vi "GS Var Common Ana Fixed Settings.vi"(1 "Action(GET)":enum16{"GET", "SET"}(ring), 7 "Common Analog Var Fixed in":T4[](array[typedef]) {"Default Scaling"."Offset" format="%.5f"; "Default Scaling"."Gain" format="%.5f"}, 9 "Common Digital Var Fixed in":T1[](array[typedef]), 11 "error in (no error)":errorcluster) -> (8 "Common Analog Var Fixed out":T4[](array[typedef]) {"Default Scaling"."Offset" format="%.5f"; "Default Scaling"."Gain" format="%.5f"}, 10 "Common Digital var Fixed":T1[](array[typedef]), 15 "error out":errorcluster)   [LabVIEW 2011]
uses:
  Fixed Analog Channel Definition.ctl
  Units/Quantity enum.ctl
  Update frequensies.ctl
  Channel catagory Enum.ctl
  Scaling.ctl
  Channel Classification Enum.ctl
  Fixed Digital Channel Definition.ctl
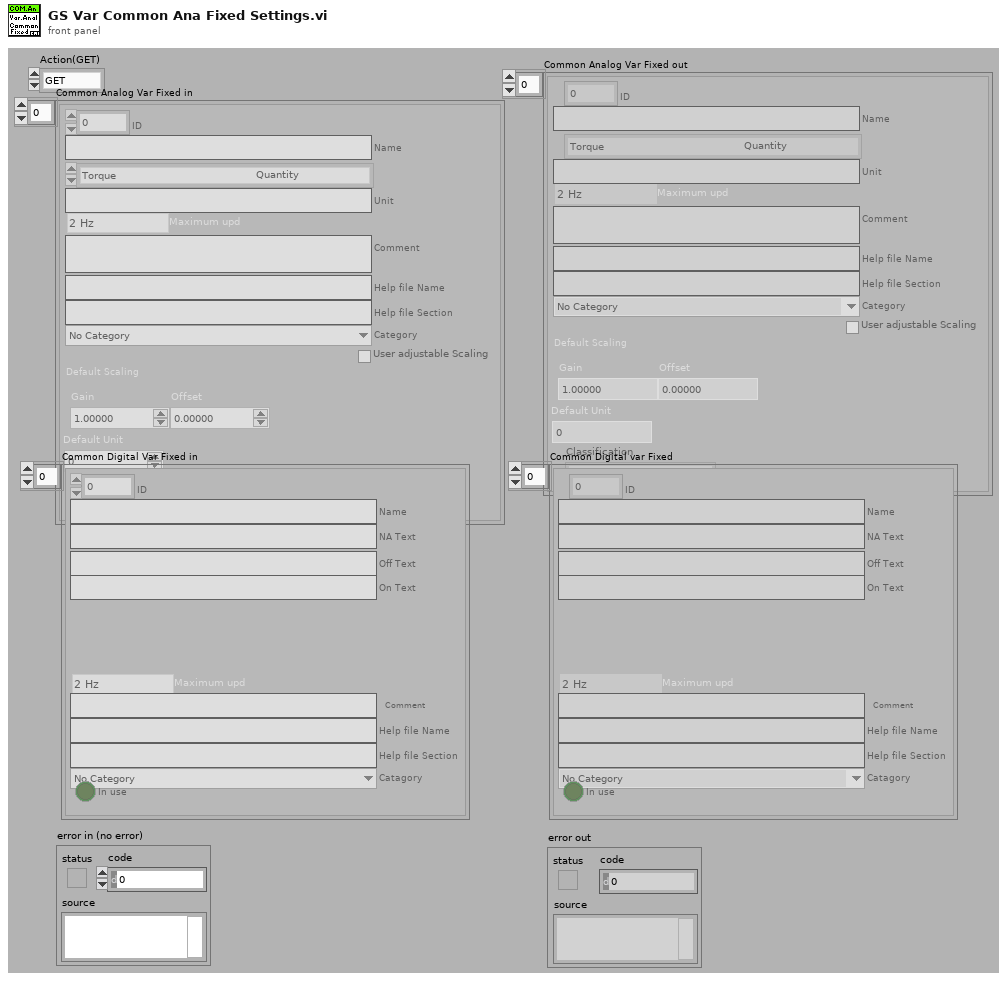
[diagram p1: front panel]
types:
  T1 = typedef "Fixed Digital Channel Definition.ctl" = cluster{"ID":u16, "Name":string, "NA Text":string, "Off Text":string, "On Text":string, "Maximum upd":T2, "Comment":string, "Help file Name":string, "Help file Section ":string, "Catagory":T3, "In use":bool}
  T2 = typedef "Update frequensies.ctl" = enum16{"2 Hz", "1 Hz", "0.1 Hz"}
  T3 = typedef "Channel catagory Enum.ctl" = enum16{"No Category", "Power", "Temperature", "Pressure"}
  T4 = typedef "Fixed Analog Channel Definition.ctl" = cluster{"ID":u16, "Name":string, "Quantity":T5, "Unit":string, "Maximum upd":T2, "Comment":string, "Help file Name":string, "Help file Section ":string, "Category":T3, "User adjustable Scaling":bool, "Default Scaling":T6, "Default Unit":i32, "Classification":T7}
  T5 = typedef "Quantity enum.ctl" = enum16{"NA", "Acceleration", "Angle", "Current", "Force", "Distance", "Pressure", "Resistance", "Rotational Speed", "Speed", "Temperature", "Tension", "Torque", "Voltage", "Weight"}
  T6 = typedef "Scaling.ctl" = cluster{"Gain":dbl, "Offset":dbl}
  T7 = typedef "Channel Classification Enum.ctl" = enum16{"Basic", "Advanced", "Expert", "Unused"}
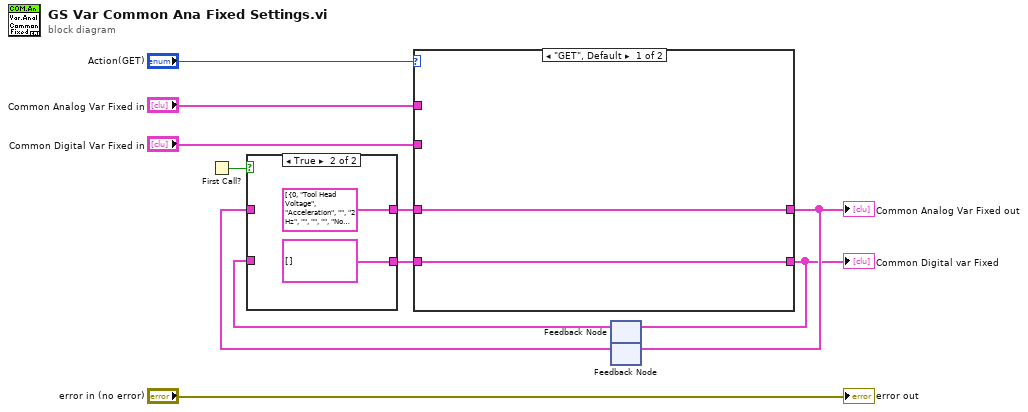
[diagram p0: block diagram]
diagram:
  n1 = First Call?() -> (First Call?: T/F=w8:bool)
  n2 = feedback #1() -> (w2:T1[])  [unwired: 1 in]
  n3 = feedback #2() -> (w9:T4[])  [unwired: 1 in]
  n4 = case shown="True" w8 {
    tunnel: w9 -> [w13 _]
    tunnel: [w13 T4[] [{"ID"=0, "Name"="Tool Head Voltage", "Quantity"=enum."Acceleration", "Unit"="", "Maximum upd"=enum."2 Hz", "Comment"="", "Help file Name"="", "Help file Section "="", "Category"=enum."No Category", "User adjustable Scaling"=FALSE, "Default Scaling"={"Gain"=0.0, "Offset"=0.0}, "Default Unit"=0, "Classification"=enum."Basic"}, {"ID"=1, "Name"="Topside Voltage", "Quantity"=enum."Acceleration", "Unit"="", "Maximum upd"=enum."2 Hz", "Comment"="", "Help file Name"="", "Help file Section "="", "Category"=enum."No Category", "User adjustable Scaling"=FALSE, "Default Scaling"={"Gain"=0.0, "Offset"=0.0}, "Default Unit"=0, "Classification"=enum."Basic"}, {"ID"=2, "Name"="Wire Current", "Quantity"=enum."Acceleration", "Unit"="", "Maximum upd"=enum."2 Hz", "Comment"="", "Help file Name"="", "Help file Section "="", "Category"=enum."No Category", "User adjustable Scaling"=FALSE, "Default Scaling"={"Gain"=0.0, "Offset"=0.0}, "Default Unit"=0, "Classification"=enum."Basic"}, {"ID"=3, "Name"="Wire Resistance", "Quantity"=enum."Acceleration", "Unit"="", "Maximum upd"=enum."2 Hz", "Comment"="", "Help file Name"="", "Help file Section "="", "Category"=enum."No Category", "User adjustable Scaling"=FALSE, "Default Scaling"={"Gain"=0.0, "Offset"=0.0}, "Default Unit"=0, "Classification"=enum."Basic"}, {"ID"=4, "Name"="Wire Length(Depth)", "Quantity"=enum."Acceleration", "Unit"="", "Maximum upd"=enum."2 Hz", "Comment"="", "Help file Name"="", "Help file Section "="", "Category"=enum."No Category", "User adjustable Scaling"=FALSE, "Default Scaling"={"Gain"=0.0, "Offset"=0.0}, "Default Unit"=0, "Classification"=enum."Basic"}, {"ID"=5, "Name"="Wire Speed", "Quantity"=enum."Acceleration", "Unit"="", "Maximum upd"=enum."2 Hz", "Comment"="", "Help file Name"="", "Help file Section "="", "Category"=enum."No Category", "User adjustable Scaling"=FALSE, "Default Scaling"={"Gain"=0.0, "Offset"=0.0}, "Default Unit"=0, "Classification"=enum."Basic"}, {"ID"=6, "Name"="Wire Tension", "Quantity"=enum."Acceleration", "Unit"="", "Maximum upd"=enum."2 Hz", "Comment"="", "Help file Name"="", "Help file Section "="", "Category"=enum."No Category", "User adjustable Scaling"=FALSE, "Default Scaling"={"Gain"=0.0, "Offset"=0.0}, "Default Unit"=0, "Classification"=enum."Basic"}] ("Common Variables Fixed")] -> w6
    tunnel: [w12 T1[] [] ("Common Variables Fixed")] -> w4
    tunnel: w2 -> [w12 _]
    frame False {
    }
    frame True {
    }
  }
  n5 = case shown="\"GET\", Default" "Action(GET)" {
    tunnel: [w17 w19] -> w7
    tunnel: w6 -> [w17 _]
    tunnel: "Common Analog Var Fixed in" -> [_ w19]
    tunnel: [w16 w18] -> w3
    tunnel: w4 -> [w16 _]
    tunnel: "Common Digital Var Fixed in" -> [_ w18]
    frame "GET", Default {
    }
    frame "SET" {
    }
  }
  "Common Analog Var Fixed out" <- w7
  "Common Digital var Fixed" <- w3
  n6 = feedback-in #1(w3) -> ()
  n7 = feedback-in #2(w7) -> ()
  "error out" <- "error in (no error)"
